vi "uni (SubVI).vi"(7 "OK Button":bool, 8 "max":dbl, 9 "min":dbl) -> (2 "maxOut":dbl, 3 "minOut":dbl)   [LabVIEW 2011]
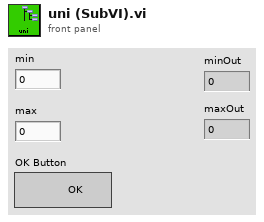
[diagram p1: front panel]
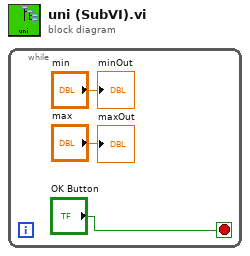
[diagram p0: block diagram]
diagram:
  n1 = while {
    stop <- "OK Button" stop-if-true
    "minOut" <- "min"
    "maxOut" <- "max"
  }
